vi "LSMcontroller_v56_from here for labview64bit.vi"() -> ()   [LabVIEW 2015] (continued)
                                n2126 = call "add channel to active arrayv2.vi"("line array in"=w5019, "line to add"=w5020) -> ("line array out"=w5018:u32[])  [unwired: 2 out]
                                n2127 = in-place-cluster #42("aDO"=w5018) -> (w5014:T12)
                                }
                                n2128 = call "2pparameters.vi"("Params in"=w5014, "command"="set") -> ()  [unwired: 1 out]
                                }
                                frame #1 {
                                n2129 = call "waveformparamsv2.vi"("command"="add DO", "add DO"=w5021) -> ()  [unwired: 3 in, 3 out]
                                }
                                frame #2 {
                                n2130 = call "waveformsDObuffer.vi"("command"="get") -> ("DO wf out"=w5026:digitalwaveform[])  [unwired: 1 in]
                                n2131 = Build Array (concatenate)(w5026, w5023) -> (w5025:digitalwaveform[])
                                n2132 = call "waveformsDObuffer.vi"("DO wf in"=w5025, "command"="set") -> ()  [unwired: 1 out]
                                }
                                }
                                }
                                frame 0 {
                                n2133 = stacked-sequence {
                                seq-local: [w5032 _ _] -> [_ w5042 w5059]
                                tunnel: w5031 -> [_ _ _]
                                tunnel: w5030 -> [_ _ _]
                                tunnel: w5029 -> [_ w5039 _]
                                tunnel: w5028 -> [_ _ w5058]
                                frame #0 {
                                n2134 = call "configuration.vi"("command"="get") -> ("config out"=w5037:T13)  [unwired: 2 in, 1 out]
                                n2135 = Unbundle By Name(w5037) -> ("LT timestamp"=w5033:u32)
                                n2136 = call "2pparameters.vi"("command"="get") -> ("params out"=w5036:T12)  [unwired: 1 in]
                                n2137 = Unbundle By Name(w5036) -> ("aDO"=w5034:u32[])
                                n2138 = Search 1D Array(1D array=w5034, element=w5033) -> (index of element=w5032:i32)  [unwired: 1 in]
                                }
                                frame #1 {
                                n2139 = local read "Measurement"() -> (w5041:T5)
                                n2140 = To Unsigned Long Integer(number=w5041) -> (unsigned 32bit integer=w5040:u32)
                                n2141 = case shown="5..7" w5040 {
                                tunnel: w5042 -> [_ w5046]
                                tunnel: w5039 -> [_ w5043]
                                frame 0..4, Default {
                                }
                                frame 5..7 {
                                n2142 = Index Array(array=w5043, index=0) -> (element=w5044:T20)
                                n2143 = call "waveformparamsv2.vi"("command"="get") -> ("Params out"=w5049:T16)  [unwired: 4 in, 2 out]
                                n2144 = in-place {
                                in-place-border: w5046 -> [w5053]
                                in-place-border: w5044 -> [w5051]
                                n2145 = in-place-cluster #43(w5049) -> ("DO parameters"=w5054:T19)
                                n2146 = in-place {
                                in-place-border: w5051 -> [w5055]
                                n2147 = in-place-array #44(w5054, w5053) -> ()  [unwired: 1 out]
                                n2148 = in-place-array #44(w5055) -> (w5052:T19)  [unwired: 1 out]
                                }
                                n2149 = in-place-cluster #43("DO parameters"=w5052) -> (w5047:T16)
                                }
                                n2150 = call "waveformparamsv2.vi"("command"="set", "Params in"=w5047) -> ()  [unwired: 3 in, 3 out]
                                }
                                }
                                }
                                frame #2 {
                                n2151 = local read "Measurement"() -> (w5057:T5)
                                n2152 = To Unsigned Long Integer(number=w5057) -> (unsigned 32bit integer=w5056:u32)
                                n2153 = case shown="5..7" w5056 {
                                tunnel: w5059 -> [_ w5063]
                                tunnel: w5058 -> [_ w5061]
                                frame 0..4, Default {
                                }
                                frame 5..7 {
                                n2154 = Index Array(array=w5061, index=0) -> (element=w5060:digitalwaveform)
                                n2155 = call "waveformsDObuffer.vi"("command"="get") -> ("DO wf out"=w5065:digitalwaveform[])  [unwired: 1 in]
                                n2156 = Replace Array Subset(array=w5065, new element=w5060, index=w5063) -> (w5067:digitalwaveform[])
                                n2157 = call "waveformsDObuffer.vi"("DO wf in"=w5067, "command"="set") -> ()  [unwired: 1 out]
                                }
                                }
                                }
                                }
                                }
                                }
                              }
                              frame #4 {
                                n2158 = call "Used AO lines.vi"() -> ("used AO names"=w5070:string[], "used AO lines"=w5068:tag[])  [unwired: 2 in]
                                n2159 = control-ref of="Analog Lines Plot"() -> (w5069:refnum<vi>)
                                n2160 = control-ref of="Digital Lines Plot"() -> (w5071:refnum<vi>)
                                n2161 = call "Used DO lines.vi"() -> ("used DO names"=w5072:string[], "used DO lines"=w5073:tag[])  [unwired: 2 in]
                                n2162 = local write "Analog Used Lines"(w5068) -> ()
                                n2163 = local write "Analog Used Names"(w5070) -> ()
                                n2164 = local write "Digital Used Lines"(w5073) -> ()
                                n2165 = local write "Digital Used Names"(w5072) -> ()
                                n2166 = call "prepDOWaveplot.vi"("DigitalGraph in"=w5071, "used DO names"=w5072) -> ()  [unwired: 1 in]
                                n2167 = call "prepAOWaveplot.vi"("WaveformGraph in"=w5069, "Analog Used Names"=w5070) -> ()  [unwired: 1 in]
                              }
                              frame #5 {
                                n2168 = local read "Meastab"() -> (w5088:enum32{"X-Y Image", "Linescan", "Timetrace"})
                                n2169 = property on="refwf" class="Ring (strict)"() -> ("RingText.Text"=w5085:string)  [unwired: 2 in, 2 out]
                                n2170 = case shown="\"Timetrace\"" w5088 {
                                tunnel: [w5090 w5091] -> w5089
                                frame "X-Y Image", Default {
                                n2171 = local read "Sampling rate"() -> (w5090:dbl)
                                }
                                frame "Timetrace" {
                                n2172 = local read "srateAODOtt"() -> (w5091:dbl)
                                }
                                }
                                n2173 = call "waveformsAObuffer.vi"("command"="get") -> ("AO wf out"=w5076:waveform(dbl)[])  [unwired: 1 in]
                                n2174 = local read "wavdet"() -> (w5086:bool)
                                n2175 = call "waveformsDObuffer.vi"("command"="get") -> ("DO wf out"=w5080:digitalwaveform[])  [unwired: 1 in]
                                n2176 = call "correctwaveformsizetemp.vi"("new sampling frequency (Hz)"=w5089, "start"=FALSE, "reference waveforms to"=w5085, "Analog waveforms in"=w5076, "stop"=TRUE, "Digital waveforms in"=w5080) -> ("analog wf out"=w5082:waveform(dbl)[], "Digital wf out"=w5084:digitalwaveform[], "measpoints"=w5087:i32)
                                n2177 = local write "Analog Lines Plot"(w5082) -> ()
                                n2178 = call "GetNumCamFramesv2.vi"("Digital Waveform Graph"=w5084) -> ("Numeric"=w5083:i32)  [unwired: 10 in]
                                n2179 = local write "Digital Lines Plot"(w5084) -> ()
                                n2180 = call "waveformsDObuffer.vi"("DO wf in"=w5084, "command"="set") -> ()  [unwired: 1 out]
                                n2181 = call "waveformsAObuffer.vi"("AO wf in"=w5082, "command"="set") -> ()  [unwired: 1 out]
                                n2182 = local write "Total Camera Frames"(w5083) -> ()
                                n2183 = case shown="True" w5086 {
                                tunnel: w5087 -> [_ w5092]
                                frame False {
                                }
                                frame True {
                                n2184 = local write "# of frames"(w5092) -> ()
                                }
                                }
                              }
                            }
                            n2185 = call "stoperaseCI.vi"() -> ()  [unwired: 12 in]
                            n2186 = call "stoperaseDO_img.vi"() -> ()  [unwired: 12 in]
                            n2187 = call "stoperaseAO_img.vi"() -> ()  [unwired: 12 in]
                            n2188 = call "stoperaseAI_img.vi"() -> ()  [unwired: 12 in]
                          }
                          frame #9 {
                            w5102 = FALSE ("Value (Signaling)")
                            n2189 = local read "save\ndata"() -> (w5097:bool)
                            n2190 = case shown="True" w5097 {
                              tunnel: w5096 -> [_ w5109]
                              frame False {
                              }
                              frame True {
                                n2191 = call "closebinaryfiles.vi"() -> ()  [unwired: 12 in]
                                n2192 = local read "filename prefix"() -> (w5111:string)
                                n2193 = local read "data dir"() -> (w5110:path)
                                n2194 = call "saveparams.vi"("timestamp"=w5109, "filename prefix in"=w5111, "data dir in"=w5110) -> ()  [unwired: 1 in]
                              }
                            }
                            n2195 = call "2pparameters.vi"("command"="get") -> ("params out"=w5093:T12)  [unwired: 1 in]
                            n2196 = Unbundle By Name(w5093) -> ("auto OD"=w5094:bool)
                            n2197 = case shown="True" w5094 {
                              frame False {
                              }
                              frame True {
                                n2198 = call "configuration.vi"("command"="get") -> ("config out"=w5105:T13)  [unwired: 2 in, 1 out]
                                n2199 = call "2pparameters.vi"("command"="get") -> ("params out"=w5108:T12)  [unwired: 1 in]
                                n2200 = Unbundle By Name(w5105) -> ("contour OD"=w5103:u16)
                                n2201 = Unbundle By Name(w5108) -> ("ODfilt"=w5104:u16)
                                n2202 = call "filterwheelcontrol_nothorlabslib.vi"("Current OD filt"=w5103, "New ODfilt"=w5104) -> ()  [unwired: 1 in]
                              }
                            }
                            n2203 = property on="Start" class="Bool (strict)"("Val(Sgnl)"=w5102) -> ()  [unwired: 2 in, 2 out]
                            n2204 = property on="Start" class="Bool (strict)"("Visible"=TRUE, "DisabledEnum"=T8."Enabled" ("Disabled")) -> ()  [unwired: 2 in, 2 out]
                            n2205 = property on="Stop" class="Bool (strict)"("Val(Sgnl)"=w5102) -> ()  [unwired: 2 in, 2 out]
                            n2206 = property on="Stop" class="Bool (strict)"("Visible"=FALSE, "DisabledEnum"=T8."Disabled" ("Disabled")) -> ()  [unwired: 2 in, 2 out]
                          }
                          frame #10 {
                            w5114 = T23 2 items=["no dialog", "OK message", "continue or stop message", "OK message + warnings", "continue/stop + warnings"] ("type of dialog (OK msg:1)")
                            n2207 = call "displayerrors.vi"() -> ("error IO"=w5115:errorcluster)
                            n2208 = call <vilib>:"General Error Handler.vi"("type of dialog (OK msg:1)"=w5114, "error in (no error)"=w5115) -> ("error out"=w5113:errorcluster)  [unwired: 9 in, 4 out]
                            n2209 = call <vilib>:"Clear Errors.vi"("error in (no error)"=w5113) -> ("error out"=w5112:errorcluster)  [unwired: 5 in, 1 out]
                            n2210 = call "seterrors.vi"("error IO"=w5112) -> ()
                          }
                        }
                      }
                    }
                  }
                  frame "Lifetime (point)" {
                    # "Disabled for conversion to 64 bit"
                    n2211 = disable-structure shown="Disabled" {
                      frame Disabled {
                        n2212 = stacked-sequence {
                          frame #0 {
                            w5126 = 12.5 ("x")
                            # "get from syncrate"
                            n2213 = local read "Bin size"() -> (w5120:T7)
                            n2214 = local read "Vx-ref"() -> (w5132:dbl)
                            n2215 = local read "Vy-ref"() -> (w5133:dbl)
                            n2216 = call "2pparameters.vi"("command"="get") -> ("params out"=w5118:T12)  [unwired: 1 in]
                            n2217 = Scale By Power Of 2(n=w5120, x=1.0 ("Y Scale.Range:Minimum")) -> (x*2^n=w5129:dbl)
                            n2218 = call "setposition.vi"("Vy"=w5133, "Vx"=w5132) -> ()  [unwired: 1 in]
                            n2219 = Unbundle By Name(w5118) -> ("autoshutter"=w5119:bool)
                            n2220 = Multiply(x=3000.0 ("Y Scale.Range:Minimum"), y=w5129) -> (x*y=w5127:dbl)
                            n2221 = Compound Arithmetic op=MULTIPLY(w5126, invert 3200.0 ("X Scale.Offset and Multiplier:Multiplier"), w5129) -> (w5128:dbl)
                            n2222 = case shown="True" w5119 {
                              frame False {
                              }
                              frame True {
                                n2223 = call "shuttercontrol.vi"("command"="open") -> ()  [unwired: 1 in, 1 out]
                              }
                            }
                            n2224 = call "lifetimeparameters.vi"("command"="get") -> ("Params out"=w5124:T21)  [unwired: 1 in]
                            n2225 = property on="Histogram" class="WFGraph (strict)"("XScale.Maximum"=w5126, "XScale.Minimum"=0.0 ("X Scale.Range:Minimum"), "YScale.Maximum"=w5127, "YScale.Minimum"=0.1 ("Y Scale.Range:Minimum"), "XScale.Multiplier"=w5128) -> ()  [unwired: 2 in, 2 out]
                            n2226 = Bundle By Name(cluster=w5124, "Bin size"=w5120) -> (w5125:T21)
                            n2227 = call "lifetimeparameters.vi"("Params in"=w5125, "command"="set") -> ()  [unwired: 1 out]
                            n2228 = property on="Histogram 2" class="WFGraph (strict)"("YScale.Maximum"=w5127, "XScale.Multiplier"=w5128, "XScale.Maximum"=w5126) -> ()  [unwired: 2 in, 2 out]
                            n2229 = call "2pparameters.vi"("command"="get") -> ("params out"=w5140:T12)  [unwired: 1 in]
                            n2230 = Bundle By Name(cluster=w5140, "type"="Lifetime (point)") -> (w5138:T12)
                            n2231 = property on="Stop" class="Bool (strict)"("Visible"=TRUE, "DisabledEnum"=T8."Enabled" ("Disabled")) -> ()  [unwired: 2 in, 2 out]
                            n2232 = property on="Start" class="Bool (strict)"("Visible"=FALSE, "DisabledEnum"=T8."Disabled and Grayed Out" ("Disabled")) -> ()  [unwired: 2 in, 2 out]
                            n2233 = call "2pparameters.vi"("Params in"=w5138, "command"="set") -> ()  [unwired: 1 out]
                          }
                          frame #1 {
                            n2234 = call "setup.vi"() -> ()  [unwired: 1 in]
                          }
                          frame #2 {
                            # "main loop"
                            n2235 = call "lifetimeparameters.vi"("command"="get") -> ("Params out"=w5150:T21)  [unwired: 1 in]
                            n2236 = Unbundle By Name(w5150) -> ("devidx"=w5148:i32)
                            n2237 = for {
                              N: 10000 -> [_]
                              tunnel: [w5151] -> w5146 mode=indexing
                              i -> [w5151]
                            }
                            n2238 = while {
                              tunnel: w5148 -> [w5155]
                              tunnel: w5146 -> [w5152]
                              i -> [w5153]
                              stop <- w5157 stop-if-true
                              n2239 = Increment(x=w5153) -> (x+1=w5154:i32)
                              n2240 = dll-call lib="phlib.dll" fn="_PH_GetCountRate@8" label="PH_GetCountRate"("devidx"=w5155, "channel"=0) -> (w5156:i32)  [unwired: 5 in, 2 out]
                              "SyncRate" <- w5156
                              n2241 = stacked-sequence {
                                seq-local: [_ _ w5164 _ _] -> [_ _ _ w5177 _]
                                seq-local: [_ _ w5163 _ _] -> [_ _ _ w5176 _]
                                seq-local: [_ w5161 _ _ _] -> [_ _ w5165 _ _]
                                tunnel: w5156 -> [_ _ _ w5184 _]
                                tunnel: w5152 -> [_ _ _ w5174 _]
                                frame #0 {
                                n2242 = call "start_binned.vi"() -> ()  [unwired: 1 in]
                                }
                                frame #1 {
                                n2243 = call "get-histogram.vi"() -> ("IntegralCount"=→"Integral count":u32, "Histogram"=w5161:u32[])
                                "Histogram" <- w5161
                                }
                                frame #2 {
                                n2244 = Search 1D Array(1D array=w5165, element=u32 0) -> (index of element=w5163:i32)  [unwired: 1 in]
                                n2245 = Multiply(x=w5163, y=0.99) -> (x*y=w5169:dbl)
                                n2246 = Array Subset(array=w5165, index=0, length=w5169) -> (w5172:u32[])
                                n2247 = Array Max & Min(array=w5172) -> (max index (indices)=w5166:i32)  [unwired: 3 out]
                                n2248 = Split 1D Array(array=w5172, index=w5166) -> (second subarray=w5168:u32[])  [unwired: 1 out]
                                n2249 = Array Max & Min(array=w5168) -> (min index (indices)=w5167:i32)  [unwired: 3 out]
                                n2250 = Split 1D Array(array=w5168, index=w5167) -> (first subarray=w5164:u32[])  [unwired: 1 out]
                                "Histogram 2" <- w5164
                                }
                                frame #3 {
                                n2251 = Array Size(array=w5177) -> (size(s)=w5179:i32)
                                n2252 = Array Subset(array=w5174, index=0, length=w5179) -> (w5178:i32[])
                                n2253 = Compound Arithmetic op=MULTIPLY(1000000000.0 ("value"), invert w5184, invert w5176, w5178) -> (w5175:dbl[])
                                n2254 = call <vilib>:"Exponential Fit.vi"("Y"=w5177, "X"=w5175) -> ("damping"=w5181:dbl)  [unwired: 8 in, 5 out]
                                n2255 = Divide(x=-1.0 ("y"), y=w5181) -> (x/y=→"Lifetime (ns)":dbl)
                                }
                                frame #4 {
                                n2256 = local read "downright"() -> (w5191:bool)
                                n2257 = local read "downleft"() -> (w5193:bool)
                                n2258 = local read "upright"() -> (w5189:bool)
                                n2259 = local read "upleft"() -> (w5187:bool)
                                n2260 = local read "down"() -> (w5192:bool)
                                n2261 = local read "right"() -> (w5190:bool)
                                n2262 = local read "left"() -> (w5194:bool)
                                n2263 = local read "up"() -> (w5188:bool)
                                n2264 = Compound Arithmetic op=OR(w5187, w5188, w5189, w5190, w5191, w5192, w5193, w5194) -> (w5186:bool)
                                n2265 = case shown="True" w5186 {
                                frame False {
                                }
                                frame True {
                                n2266 = stacked-sequence {
                                frame #0 {
                                n2267 = local read "downright"() -> (w5196:bool)
                                n2268 = local read "downleft"() -> (w5198:bool)
                                n2269 = local read "BigSmall"() -> (w5195:bool)
                                n2270 = local read "upright"() -> (w5200:bool)
                                n2271 = local read "upleft"() -> (w5203:bool)
                                n2272 = local read "down"() -> (w5199:bool)
                                n2273 = local read "right"() -> (w5201:bool)
                                n2274 = local read "left"() -> (w5197:bool)
                                n2275 = local read "up"() -> (w5202:bool)
                                n2276 = call "movestageparams.vi"("command"="get") -> ("Params out"=w5206:T22)  [unwired: 1 in]
                                n2277 = Bundle By Name(cluster=w5206, "upleft"=w5203, "up"=w5202, "upright"=w5200, "right"=w5201, "downright"=w5196, "down"=w5199, "downleft"=w5198, "left"=w5197, "Bigsmall"=w5195) -> (w5207:T22)
                                n2278 = call "movestageparams.vi"("Params in"=w5207, "command"="set") -> ()  [unwired: 1 out]
                                }
                                frame #1 {
                                n2279 = call "movestage.vi"() -> ()  [unwired: 12 in]
                                }
                                frame #2 {
                                w5208 = FALSE ("OK Button")
                                w5209 = FALSE ("OK Button")
                                n2280 = property on="down" class="Bool (strict)"("Value"=w5209) -> ()  [unwired: 2 in, 2 out]
                                n2281 = property on="up" class="Bool (strict)"("Value"=w5209) -> ()  [unwired: 2 in, 2 out]
                                n2282 = property on="right" class="Bool (strict)"("Value"=w5209) -> ()  [unwired: 2 in, 2 out]
                                n2283 = property on="left" class="Bool (strict)"("Value"=w5209) -> ()  [unwired: 2 in, 2 out]
                                n2284 = property on="upleft" class="Bool (strict)"("Value"=w5208) -> ()  [unwired: 2 in, 2 out]
                                n2285 = property on="upright" class="Bool (strict)"("Value"=w5208) -> ()  [unwired: 2 in, 2 out]
                                n2286 = property on="downleft" class="Bool (strict)"("Value"=w5208) -> ()  [unwired: 2 in, 2 out]
                                n2287 = property on="downright" class="Bool (strict)"("Value"=w5208) -> ()  [unwired: 2 in, 2 out]
                                }
                                }
                                }
                                }
                                }
                              }
                              n2288 = dll-call lib="phlib.dll" fn="_PH_GetCountRate@8" label="PH_GetCountRate"("devidx"=w5155, "channel"=1) -> (→"Ch1Rate":i32)  [unwired: 5 in, 2 out]
                              n2289 = local read "Stop"() -> (w5157:bool)
                              n2290 = local write "points recorded"(w5154) -> ()
                            }
                          }
                          frame #3 {
                            w5217 = FALSE ("Value (Signaling)")
                            n2291 = call "2pparameters.vi"("command"="get") -> ("params out"=w5211:T12)  [unwired: 1 in]
                            n2292 = Unbundle By Name(w5211) -> ("autoshutter"=w5212:bool)
                            n2293 = case shown="True" w5212 {
                              frame False {
                              }
                              frame True {
                                n2294 = call "shuttercontrol.vi"("command"="close") -> ()  [unwired: 1 in, 1 out]
                              }
                            }
                            n2295 = property on="Start" class="Bool (strict)"("Val(Sgnl)"=w5217) -> ()  [unwired: 2 in, 2 out]
                            n2296 = property on="Start" class="Bool (strict)"("Visible"=TRUE, "DisabledEnum"=T8."Enabled" ("Disabled")) -> ()  [unwired: 2 in, 2 out]
                            n2297 = property on="Stop" class="Bool (strict)"("Val(Sgnl)"=w5217) -> ()  [unwired: 2 in, 2 out]
                            n2298 = property on="Stop" class="Bool (strict)"("Visible"=FALSE, "DisabledEnum"=T8."Disabled" ("Disabled")) -> ()  [unwired: 2 in, 2 out]
                          }
                        }
                      }
                      frame Enabled {
                      }
                    }
                    n2299 = local write "64bit disabled"(TRUE ("64bit disabled")) -> ()
                  }
                }
              }
            }
          }
          event "avpp", "Angle ref", "xpixels ref", "Vx-min ref", "Vx-max ref", "ypixels ref", "Vy-min ref", "Vy-max ref", "ROI Type", "Sampling rate": Value Change {
            n2300 = event-data() -> ()  [unwired: 1 in, 6 out]
            n2301 = local read "avpp"() -> (w5236:i32)
            n2302 = local read "Angle ref"() -> (w5235:dbl)
            n2303 = local read "ROI Type"() -> (w5234:u16)
            n2304 = local read "xpixels ref"() -> (w5231:i32)
            n2305 = local read "Vx-min ref"() -> (w5230:dbl)
            n2306 = local read "Vx-max ref"() -> (w5229:dbl)
            n2307 = local read "ypixels ref"() -> (w5227:i32)
            n2308 = local read "Vy-min ref"() -> (w5228:dbl)
            n2309 = local read "Vy-max ref"() -> (w5224:dbl)
            n2310 = local read "Sampling rate"() -> (w5219:dbl)
            n2311 = local read "# of frames"() -> (w5223:i32)
            n2312 = local read "maxbufferAI"() -> (w5222:i32)
            n2313 = local read "Override AI buffer"() -> (w5220:bool)
            n2314 = call "2pparameters.vi"("command"="get") -> ("params out"=w5233:T12)  [unwired: 1 in]
            n2315 = Bundle By Name(cluster=w5233, "avpp"=w5236, "Angle Img"=w5235, "Xpixels Img"=w5231, "Vx-min Img"=w5230, "VX-max Img"=w5229, "Ypixels Img"=w5227, "Vy-min Img"=w5228, "Vy-max Img"=w5224, "srate"=w5219, "srate Img"=w5219, "measpoints"=w5223, "maxbufferAI"=w5222, "Drawing Mode"=w5234, "Vz-reset"=0.0, "AIoverride"=w5220) -> (w5225:T12)
            n2316 = call "2pparameters.vi"("Params in"=w5225, "command"="set") -> ()  [unwired: 1 out]
          }
          event "# of frames": Value Change {
            n2317 = event-data() -> ()  [unwired: 1 in, 6 out]
            n2318 = local read "Meastab"() -> (w5237:enum32{"X-Y Image", "Linescan", "Timetrace"})
            n2319 = case shown="\"X-Y Image\", Default" w5237 {
              frame "X-Y Image", Default {
                n2320 = local read "# of frames"() -> (w5238:i32)
                n2321 = call "2pparameters.vi"("command"="get") -> ("params out"=w5242:T12)  [unwired: 1 in]
                n2322 = Bundle By Name(cluster=w5242, "measpoints"=w5238) -> (w5239:T12)
                n2323 = call "2pparameters.vi"("Params in"=w5239, "command"="set") -> ()  [unwired: 1 out]
              }
              frame "Linescan" {
                n2324 = local read "srateAODOtt"() -> (w5252:dbl)
                n2325 = local read "# of frames"() -> (w5248:i32)
                n2326 = local read "refreshtime"() -> (w5254:dbl)
                n2327 = local read "bin"() -> (w5249:dbl)
                n2328 = call "tt_timeandsamples.vi"("bin"=w5249, "refreshtime"=w5254, "srateAODOtt"=w5252, "tot#ofsamples"=w5248) -> ("refreshrate"=w5251:dbl, "refreshbuffer"=w5250:i32, "timetracecycles"=w5247:i32)  [unwired: 5 in]
                n2329 = call "2pparameters.vi"("command"="get") -> ("params out"=w5244:T12)  [unwired: 1 in]
                n2330 = Bundle By Name(cluster=w5244, "measpoints"=w5248, "tt_cycles"=w5247, "refreshbuffer"=w5250, "refreshrate"=w5251) -> (w5246:T12)
                n2331 = Reciprocal(x=w5251) -> (1/x=w5253:dbl)
                n2332 = local write "refreshtime"(w5253) -> ()
                n2333 = call "2pparameters.vi"("Params in"=w5246, "command"="set") -> ()  [unwired: 1 out]
              }
              frame "Timetrace" {
                n2334 = local read "srateAODOtt"() -> (w5264:dbl)
                n2335 = local read "# of frames"() -> (w5260:i32)
                n2336 = local read "refreshtime"() -> (w5266:dbl)
                n2337 = local read "bin"() -> (w5261:dbl)
                n2338 = call "tt_timeandsamples.vi"("bin"=w5261, "refreshtime"=w5266, "srateAODOtt"=w5264, "tot#ofsamples"=w5260) -> ("refreshrate"=w5263:dbl, "refreshbuffer"=w5262:i32, "timetracecycles"=w5259:i32)  [unwired: 5 in]
                n2339 = call "2pparameters.vi"("command"="get") -> ("params out"=w5256:T12)  [unwired: 1 in]
                n2340 = Bundle By Name(cluster=w5256, "measpoints"=w5260, "tt_cycles"=w5259, "refreshbuffer"=w5262, "refreshrate"=w5263) -> (w5258:T12)
                n2341 = Reciprocal(x=w5263) -> (1/x=w5265:dbl)
                n2342 = local write "refreshtime"(w5265) -> ()
                n2343 = call "2pparameters.vi"("Params in"=w5258, "command"="set") -> ()  [unwired: 1 out]
              }
            }
          }
          event "srateAODOtt", "refreshtime", "Vx-ref", "Vy-ref", "Vx-min draw", "Vx-max draw", "Vy-min draw", "Vy-max draw", "bin": Value Change {
            n2344 = event-data() -> ()  [unwired: 1 in, 6 out]
            n2345 = local read "ypixels ref"() -> (w5298:i32)
            n2346 = local read "Vy-min draw"() -> (w5274:dbl)
            n2347 = local read "Vy-max draw"() -> (w5273:dbl)
            n2348 = local read "Vx-min draw"() -> (w5276:dbl)
            n2349 = local read "Vx-max draw"() -> (w5275:dbl)
            n2350 = local read "xpixels ref"() -> (w5272:i32)
            n2351 = local read "ROI Type"() -> (w5271:u16)
            n2352 = local read "Pel"() -> (w5270:dbl)
            n2353 = local read "srateAODOtt"() -> (w5280:dbl)
            n2354 = local read "# of frames"() -> (w5285:i32)
            n2355 = local read "refreshtime"() -> (w5278:dbl)
            n2356 = local read "bin"() -> (w5283:dbl)
            n2357 = local read "Override AI buffer"() -> (w5268:bool)
            n2358 = local read "finite samples"() -> (w5292:bool)
            n2359 = local read "srateAODOtt"() -> (w5267:dbl)
            n2360 = local read "srateAODOtt"() -> (w5286:dbl)
            n2361 = local read "continuous"() -> (w5291:bool)
            n2362 = local read "Angle ref"() -> (w5277:dbl)
            n2363 = local read "wavdet"() -> (w5293:bool)
            n2364 = local read "Vx-ref"() -> (w5288:dbl)
            n2365 = local read "Vy-ref"() -> (w5290:dbl)
            n2366 = local read "avpp"() -> (w5289:i32)
            n2367 = call "tt_timeandsamples.vi"("bin"=w5283, "refreshtime"=w5278, "srateAODOtt"=w5280, "tot#ofsamples"=w5285) -> ("refreshrate"=w5281:dbl, "refreshbuffer"=w5282:i32, "timetracecycles"=w5287:i32)  [unwired: 5 in]
            n2368 = local read "bin"() -> (w5284:dbl)
            n2369 = call "2pparameters.vi"("command"="get") -> ("params out"=w5296:T12)  [unwired: 1 in]
            n2370 = Bundle By Name(cluster=w5296, "Drawing Mode"=w5271, "measpoints"=w5285, "tt_cycles"=w5287, "refreshbuffer"=w5282, "refreshrate"=w5281, "Vx-ref"=w5288, "Vy-ref"=w5290, "srate"=w5267, "finite"=w5292, "cont"=w5291, "wavdet"=w5293, "avpp"=w5289, "srateAODO"=w5286, "bufferAI"=w5282, "bin"=w5284, "Angle Img"=w5277, "Vxminref"=w5276, "Vxmaxref"=w5275, "Vyminref"=w5274, "Vymaxref"=w5273, "Xpixels Img"=w5272, "Ypixels Img"=w5298, "Pel"=w5270, "Vz-reset"=0.0, "AIoverride"=w5268) -> (w5294:T12)
            n2371 = Reciprocal(x=w5281) -> (1/x=w5279:dbl)
            n2372 = local write "refreshtime"(w5279) -> ()
            n2373 = call "2pparameters.vi"("Params in"=w5294, "command"="set") -> ()  [unwired: 1 out]
          }
          event "Init": Value Change {
            # "Disabled for conversion to 64 bit"
            n2374 = event-data() -> ()  [unwired: 1 in, 6 out]
            n2375 = disable-structure shown="Disabled" {
              frame Disabled {
                n2376 = flat-sequence {
                  frame #0 {
                    n2377 = local read "Measurement"() -> (w5300:T5)
                    n2378 = case shown="\"Lifetime (scan)\", \"Lifetime (contour)\"" w5300 {
                      frame "X-Y-t movie", Default {
                      }
                      frame "Lifetime (point)" {
                        n2379 = stacked-sequence {
                          frame #0 {
                            n2380 = call "initialize.vi"("mode"=0) -> ()
                          }
                          frame #1 {
                            n2381 = call "calib.vi"() -> ()  [unwired: 1 in]
                          }
                        }
                      }
                      frame "Lifetime (scan)", "Lifetime (contour)" {
                        n2382 = stacked-sequence {
                          frame #0 {
                            n2383 = call "initialize.vi"("mode"=3) -> ()
                          }
                          frame #1 {
                            n2384 = call "calib.vi"() -> ()  [unwired: 1 in]
                          }
                        }
                      }
                    }
                  }
                  frame #1 {
                    n2385 = property on="Start" class="Bool (strict)"("Visible"=TRUE, "DisabledEnum"=T8."Enabled" ("Disabled")) -> ()  [unwired: 2 in, 2 out]
                    n2386 = property on="Init" class="Bool (strict)"("Visible"=FALSE, "DisabledEnum"=T8."Disabled and Grayed Out" ("Disabled"), "Value"=FALSE ("Init")) -> ()  [unwired: 2 in, 2 out]
                  }
                }
              }
              frame Enabled {
              }
            }
            n2387 = local write "64bit disabled"(TRUE ("64bit disabled")) -> ()
          }
          event "Measurement": Value Change {
            n2388 = event-data() -> ()  [unwired: 1 in, 5 out]
            n2389 = case shown="\"Lifetime (contour)\"" "Measurement" {
              frame "X-Y-t movie" {
                w5310 = T8."Disabled" ("Disabled")
                w5309 = FALSE ("Visible")
                n2390 = call "2pparameters.vi"("command"="get") -> ("params out"=w5320:T12)  [unwired: 1 in]
                n2391 = local write "graphtab"(T6."image" ("graphtab")) -> ()
                n2392 = local write "Save tab"(enum32{"withsave", "withoutsave"}."withsave" ("Save tab")) -> ()
                n2393 = Bundle By Name(cluster=w5320, "type"="X-Y-t movie") -> (w5318:T12)
                n2394 = call "2pparameters.vi"("Params in"=w5318, "command"="set") -> ()  [unwired: 1 out]
                n2395 = property on="refreshtime" class="DigNum (strict)"("Visible"=FALSE, "DisabledEnum"=T8."Disabled and Grayed Out" ("Disabled")) -> ()  [unwired: 2 in, 2 out]
                n2396 = property on="ttt" class="Enum (strict)"("Visible"=FALSE) -> ()  [unwired: 2 in, 2 out]
                n2397 = property on="# of frames" class="DigNum (strict)"("DisabledEnum"=T8."Enabled" ("Disabled"), "Caption.Text"="# of frames") -> ()  [unwired: 2 in, 2 out]
                n2398 = property on="continuous" class="Bool (strict)"("Visible"=TRUE, "DisabledEnum"=T8."Enabled" ("Disabled")) -> ()  [unwired: 2 in, 2 out]
                n2399 = property on="finite samples" class="Bool (strict)"("Visible"=TRUE, "DisabledEnum"=T8."Enabled" ("Disabled")) -> ()  [unwired: 2 in, 2 out]
                n2400 = property on="avpp" class="DigNum (strict)"("Visible"=TRUE, "DisabledEnum"=T8."Enabled" ("Disabled")) -> ()  [unwired: 2 in, 2 out]
                n2401 = property on="srateAODOtt" class="DigNum (strict)"("Visible"=FALSE, "DisabledEnum"=T8."Disabled" ("Disabled")) -> ()  [unwired: 2 in, 2 out]
                n2402 = local write "save\ndata"(TRUE ("save\ndata")) -> ()
                n2403 = property on="finite samples" class="Bool (strict)"("Val(Sgnl)"=TRUE ("continuous for display")) -> ()  [unwired: 2 in, 2 out]
                n2404 = property on="continuous" class="Bool (strict)"("Value"=FALSE ("continuous for display")) -> ()  [unwired: 2 in, 2 out]
                n2405 = property on="Current Average" class="DigNum (strict)"("Visible"=TRUE, "DisabledEnum"=T8."Enabled" ("Disabled")) -> ()  [unwired: 2 in, 2 out]
                n2406 = property on="img_CH1" class="IntGraph (strict)"("ZScale.Maximum"=7.0 ("Z Scale.Range:Maximum")) -> ()  [unwired: 2 in, 2 out]
                n2407 = property on="Sampling rate" class="DigNum (strict)"("Visible"=TRUE, "DisabledEnum"=T8."Enabled" ("Disabled")) -> ()  [unwired: 2 in, 2 out]
                n2408 = property on="Pel" class="DigNum (strict)"("Visible"=w5309, "DisabledEnum"=w5310) -> ()  [unwired: 2 in, 2 out]
                n2409 = property on="bin" class="DigNum (strict)"("Visible"=w5309, "DisabledEnum"=w5310) -> ()  [unwired: 2 in, 2 out]
                "Meastab" <- enum32{"X-Y Image", "Linescan", "Timetrace"}."X-Y Image" ("Meastab")
                "Zscantab" <- enum32{"withzscan", "withoutzscan", "lifetime"}."withoutzscan" ("Zscantab")
              }
              frame "X-Y-Z stack" {
                w5342 = T8."Disabled" ("Disabled")
                w5341 = FALSE ("Visible")
                n2410 = call "2pparameters.vi"("command"="get") -> ("params out"=w5352:T12)  [unwired: 1 in]
                n2411 = call "2pparameters.vi"("command"="get") -> ("params out"=w5356:T12)  [unwired: 1 in]
                n2412 = Bundle By Name(cluster=w5352, "type"="X-Y-Z stack") -> (w5350:T12)
                n2413 = Unbundle By Name(w5356) -> ("motorref"=w5355:refnum<k7>)
                n2414 = call "2pparameters.vi"("Params in"=w5350, "command"="set") -> ()  [unwired: 1 out]
                n2415 = local write "Zscantab"(enum32{"withzscan", "withoutzscan", "lifetime"}."withzscan" ("Zscantab")) -> ()
                n2416 = local write "Meastab"(enum32{"X-Y Image", "Linescan", "Timetrace"}."X-Y Image" ("Meastab")) -> ()
                n2417 = invoke class="MG17Motor" method="GetPosition"(reference=w5355, "lChanID"=0, "pfPosition"=sgl 0.0) -> ("pfPosition"=w5367:sgl)  [unwired: 2 in, 4 out]
                n2418 = property on="refreshtime" class="DigNum (strict)"("Visible"=FALSE, "DisabledEnum"=T8."Disabled and Grayed Out" ("Disabled")) -> ()  [unwired: 2 in, 2 out]
                n2419 = property on="ttt" class="Enum (strict)"("Visible"=FALSE) -> ()  [unwired: 2 in, 2 out]
                n2420 = Multiply(x=w5367, y=1000.0) -> (x*y=w5366:dbl)
                n2421 = local write "Actual Z position"(w5366) -> ()
                n2422 = local write "Save tab"(enum32{"withsave", "withoutsave"}."withsave" ("Save tab")) -> ()
                n2423 = property on="finite samples" class="Bool (strict)"("Visible"=FALSE, "DisabledEnum"=T8."Disabled and Grayed Out" ("Disabled")) -> ()  [unwired: 2 in, 2 out]
                n2424 = property on="avpp" class="DigNum (strict)"("Visible"=TRUE, "DisabledEnum"=T8."Enabled" ("Disabled")) -> ()  [unwired: 2 in, 2 out]
                n2425 = property on="continuous" class="Bool (strict)"("Visible"=FALSE, "DisabledEnum"=T8."Disabled and Grayed Out" ("Disabled")) -> ()  [unwired: 2 in, 2 out]
                n2426 = property on="img_CH1" class="IntGraph (strict)"("ZScale.Maximum"=7.0 ("Z Scale.Range:Maximum")) -> ()  [unwired: 2 in, 2 out]
                n2427 = property on="srateAODOtt" class="DigNum (strict)"("Visible"=FALSE, "DisabledEnum"=T8."Disabled" ("Disabled")) -> ()  [unwired: 2 in, 2 out]
                n2428 = property on="Pel" class="DigNum (strict)"("Visible"=w5341, "DisabledEnum"=w5342) -> ()  [unwired: 2 in, 2 out]
                n2429 = property on="bin" class="DigNum (strict)"("Visible"=w5341, "DisabledEnum"=w5342) -> ()  [unwired: 2 in, 2 out]
                n2430 = property on="Current Average" class="DigNum (strict)"("Visible"=TRUE, "DisabledEnum"=T8."Enabled" ("Disabled")) -> ()  [unwired: 2 in, 2 out]
                n2431 = property on="# of frames" class="DigNum (strict)"("Caption.Text"="# of slices", "DisabledEnum"=T8."Disabled and Grayed Out" ("Disabled")) -> ()  [unwired: 2 in, 2 out]
                n2432 = local write "save\ndata"(TRUE ("save\ndata")) -> ()
                n2433 = property on="finite samples" class="Bool (strict)"("Val(Sgnl)"=TRUE ("continuous for display")) -> ()  [unwired: 2 in, 2 out]
                n2434 = property on="continuous" class="Bool (strict)"("Value"=FALSE ("continuous for display")) -> ()  [unwired: 2 in, 2 out]
                n2435 = property on="Sampling rate" class="DigNum (strict)"("Visible"=TRUE, "DisabledEnum"=T8."Enabled" ("Disabled")) -> ()  [unwired: 2 in, 2 out]
              }
              frame "X-Y-Z-t movie" {
                w5381 = T8."Disabled" ("Disabled")
                w5380 = FALSE ("Visible")
                n2436 = property on="# of frames" class="DigNum (strict)"("DisabledEnum"=T8."Enabled" ("Disabled")) -> ()  [unwired: 2 in, 2 out]
                n2437 = property on="Current Average" class="DigNum (strict)"("Visible"=TRUE, "DisabledEnum"=T8."Enabled" ("Disabled")) -> ()  [unwired: 2 in, 2 out]
                n2438 = property on="avpp" class="DigNum (strict)"("Visible"=TRUE, "DisabledEnum"=T8."Enabled" ("Disabled")) -> ()  [unwired: 2 in, 2 out]
                n2439 = local write "Save tab"(enum32{"withsave", "withoutsave"}."withsave" ("Save tab")) -> ()
                n2440 = local write "Zscantab"(enum32{"withzscan", "withoutzscan", "lifetime"}."withzscan" ("Zscantab")) -> ()
                n2441 = local write "Meastab"(enum32{"X-Y Image", "Linescan", "Timetrace"}."X-Y Image" ("Meastab")) -> ()
                n2442 = property on="refreshtime" class="DigNum (strict)"("Visible"=FALSE, "DisabledEnum"=T8."Disabled and Grayed Out" ("Disabled")) -> ()  [unwired: 2 in, 2 out]
                n2443 = property on="ttt" class="Enum (strict)"("Visible"=FALSE) -> ()  [unwired: 2 in, 2 out]
                n2444 = call "2pparameters.vi"("command"="get") -> ("params out"=w5391:T12)  [unwired: 1 in]
                n2445 = Bundle By Name(cluster=w5391, "type"="X-Y-Z-t movie") -> (w5389:T12)
                n2446 = property on="continuous" class="Bool (strict)"("Visible"=TRUE, "DisabledEnum"=T8."Enabled" ("Disabled")) -> ()  [unwired: 2 in, 2 out]
                n2447 = property on="finite samples" class="Bool (strict)"("Visible"=TRUE, "DisabledEnum"=T8."Enabled" ("Disabled")) -> ()  [unwired: 2 in, 2 out]
                n2448 = call "2pparameters.vi"("Params in"=w5389, "command"="set") -> ()  [unwired: 1 out]
                n2449 = property on="srateAODOtt" class="DigNum (strict)"("Visible"=FALSE, "DisabledEnum"=T8."Disabled" ("Disabled")) -> ()  [unwired: 2 in, 2 out]
                n2450 = local write "save\ndata"(TRUE ("save\ndata")) -> ()
                n2451 = property on="img_CH1" class="IntGraph (strict)"("ZScale.Maximum"=7.0 ("Z Scale.Range:Maximum")) -> ()  [unwired: 2 in, 2 out]
                n2452 = property on="continuous" class="Bool (strict)"("Value"=FALSE ("continuous for display")) -> ()  [unwired: 2 in, 2 out]
                n2453 = property on="finite samples" class="Bool (strict)"("Value"=TRUE ("continuous for display")) -> ()  [unwired: 2 in, 2 out]
                n2454 = property on="Sampling rate" class="DigNum (strict)"("Visible"=TRUE, "DisabledEnum"=T8."Enabled" ("Disabled")) -> ()  [unwired: 2 in, 2 out]
                n2455 = property on="Pel" class="DigNum (strict)"("Visible"=w5380, "DisabledEnum"=w5381) -> ()  [unwired: 2 in, 2 out]
                n2456 = property on="bin" class="DigNum (strict)"("Visible"=w5380, "DisabledEnum"=w5381) -> ()  [unwired: 2 in, 2 out]
              }
              frame "linescan" {
                w5411 = T8."Enabled" ("Disabled")
                w5410 = TRUE ("Visible")
                w5413 = T8."Enabled" ("Disabled")
                w5412 = TRUE ("Visible")
                n2457 = local write "Meastab"(enum32{"X-Y Image", "Linescan", "Timetrace"}."Linescan" ("Meastab")) -> ()
                n2458 = property on="Current Average" class="DigNum (strict)"("Visible"=TRUE, "DisabledEnum"=T8."Enabled" ("Disabled")) -> ()  [unwired: 2 in, 2 out]
                n2459 = local write "Save tab"(enum32{"withsave", "withoutsave"}."withsave" ("Save tab")) -> ()
                n2460 = local write "Zscantab"(enum32{"withzscan", "withoutzscan", "lifetime"}."withoutzscan" ("Zscantab")) -> ()
                n2461 = property on="refreshtime" class="DigNum (strict)"("Visible"=FALSE, "DisabledEnum"=T8."Disabled and Grayed Out" ("Disabled")) -> ()  [unwired: 2 in, 2 out]
                n2462 = property on="continuous" class="Bool (strict)"("Value"=FALSE ("continuous for display")) -> ()  [unwired: 2 in, 2 out]
                n2463 = property on="finite samples" class="Bool (strict)"("Value"=TRUE ("continuous for display")) -> ()  [unwired: 2 in, 2 out]
                n2464 = property on="ttt" class="Enum (strict)"("Visible"=FALSE) -> ()  [unwired: 2 in, 2 out]
                n2465 = local write "save\ndata"(TRUE ("save\ndata")) -> ()
                n2466 = call "2pparameters.vi"("command"="get") -> ("params out"=w5422:T12)  [unwired: 1 in]
                n2467 = Bundle By Name(cluster=w5422, "type"="linescan") -> (w5420:T12)
                n2468 = property on="# of frames" class="DigNum (strict)"("DisabledEnum"=T8."Enabled" ("Disabled"), "Caption.Text"="# of lines") -> ()  [unwired: 2 in, 2 out]
                n2469 = property on="continuous" class="Bool (strict)"("Visible"=TRUE, "DisabledEnum"=T8."Enabled" ("Disabled")) -> ()  [unwired: 2 in, 2 out]
                n2470 = property on="avpp" class="DigNum (strict)"("Visible"=TRUE, "DisabledEnum"=T8."Enabled" ("Disabled")) -> ()  [unwired: 2 in, 2 out]
                n2471 = property on="finite samples" class="Bool (strict)"("Visible"=TRUE, "DisabledEnum"=T8."Enabled" ("Disabled")) -> ()  [unwired: 2 in, 2 out]
                n2472 = property on="srateAODOtt" class="DigNum (strict)"("Visible"=TRUE, "DisabledEnum"=T8."Enabled" ("Disabled")) -> ()  [unwired: 2 in, 2 out]
                n2473 = call "2pparameters.vi"("Params in"=w5420, "command"="set") -> ()  [unwired: 1 out]
                n2474 = property on="Pel" class="DigNum (strict)"("Visible"=w5412, "DisabledEnum"=w5413) -> ()  [unwired: 2 in, 2 out]
                n2475 = property on="bin" class="DigNum (strict)"("Visible"=w5412, "DisabledEnum"=w5413) -> ()  [unwired: 2 in, 2 out]
                n2476 = property on="Sampling rate" class="DigNum (strict)"("Visible"=FALSE, "DisabledEnum"=T8."Disabled" ("Disabled")) -> ()  [unwired: 2 in, 2 out]
                n2477 = property on="Pel" class="DigNum (strict)"("Visible"=w5410, "DisabledEnum"=w5411) -> ()  [unwired: 2 in, 2 out]
                n2478 = property on="bin" class="DigNum (strict)"("Visible"=w5410, "DisabledEnum"=w5411) -> ()  [unwired: 2 in, 2 out]
              }
              frame "Timetrace" {
                w5443 = T8."Enabled" ("Disabled")
                w5442 = TRUE ("Visible")
                n2479 = call "2pparameters.vi"("command"="get") -> ("params out"=w5448:T12)  [unwired: 1 in]
                n2480 = local write "Meastab"(enum32{"X-Y Image", "Linescan", "Timetrace"}."Timetrace" ("Meastab")) -> ()
                n2481 = Unbundle By Name(w5448) -> ("Angle draw"=w5450:dbl)
                n2482 = local write "Zscantab"(enum32{"withzscan", "withoutzscan", "lifetime"}."withoutzscan" ("Zscantab")) -> ()
                n2483 = property on="# of frames" class="DigNum (strict)"("DisabledEnum"=T8."Enabled" ("Disabled"), "Caption.Text"="# of samples") -> ()  [unwired: 2 in, 2 out]
                n2484 = property on="refreshtime" class="DigNum (strict)"("Visible"=TRUE, "DisabledEnum"=T8."Enabled" ("Disabled")) -> ()  [unwired: 2 in, 2 out]
                n2485 = property on="avpp" class="DigNum (strict)"("Visible"=FALSE, "DisabledEnum"=T8."Disabled and Grayed Out" ("Disabled")) -> ()  [unwired: 2 in, 2 out]
                n2486 = property on="Current Average" class="DigNum (strict)"("Visible"=FALSE, "DisabledEnum"=T8."Disabled and Grayed Out" ("Disabled")) -> ()  [unwired: 2 in, 2 out]
                n2487 = local write "Angle drawing"(w5450) -> ()
                n2488 = property on="ttt" class="Enum (strict)"("Visible"=TRUE) -> ()  [unwired: 2 in, 2 out]
                n2489 = property on="continuous" class="Bool (strict)"("Visible"=TRUE, "DisabledEnum"=T8."Enabled" ("Disabled")) -> ()  [unwired: 2 in, 2 out]
                n2490 = property on="finite samples" class="Bool (strict)"("Visible"=TRUE, "DisabledEnum"=T8."Enabled" ("Disabled")) -> ()  [unwired: 2 in, 2 out]
                n2491 = local write "save\ndata"(TRUE ("save\ndata")) -> ()
                n2492 = property on="finite samples" class="Bool (strict)"("Val(Sgnl)"=TRUE ("continuous for display")) -> ()  [unwired: 2 in, 2 out]
                n2493 = property on="continuous" class="Bool (strict)"("Value"=FALSE ("continuous for display")) -> ()  [unwired: 2 in, 2 out]
                n2494 = local write "Save tab"(enum32{"withsave", "withoutsave"}."withsave" ("Save tab")) -> ()
                n2495 = property on="srateAODOtt" class="DigNum (strict)"("Visible"=TRUE, "DisabledEnum"=T8."Enabled" ("Disabled")) -> ()  [unwired: 2 in, 2 out]
                n2496 = call "2pparameters.vi"("command"="get") -> ("params out"=w5455:T12)  [unwired: 1 in]
                n2497 = Bundle By Name(cluster=w5455, "type"="Timetrace") -> (w5453:T12)
                n2498 = property on="Sampling rate" class="DigNum (strict)"("Visible"=FALSE, "DisabledEnum"=T8."Disabled" ("Disabled")) -> ()  [unwired: 2 in, 2 out]
                n2499 = property on="Pel" class="DigNum (strict)"("Visible"=w5442, "DisabledEnum"=w5443) -> ()  [unwired: 2 in, 2 out]
                n2500 = property on="bin" class="DigNum (strict)"("Visible"=w5442, "DisabledEnum"=w5443) -> ()  [unwired: 2 in, 2 out]
                n2501 = call "2pparameters.vi"("Params in"=w5453, "command"="set") -> ()  [unwired: 1 out]
              }
              frame "Lifetime (point)" {
                w5476 = T8."Enabled" ("Disabled")
                w5475 = TRUE ("Visible")
                n2502 = property on="Pel" class="DigNum (strict)"("Visible"=w5475, "DisabledEnum"=w5476) -> ()  [unwired: 2 in, 2 out]
                n2503 = property on="bin" class="DigNum (strict)"("Visible"=w5475, "DisabledEnum"=w5476) -> ()  [unwired: 2 in, 2 out]
                n2504 = property on="ttt" class="Enum (strict)"("Visible"=FALSE) -> ()  [unwired: 2 in, 2 out]
                n2505 = local write "Zscantab"(enum32{"withzscan", "withoutzscan", "lifetime"}."lifetime" ("Zscantab")) -> ()
                n2506 = local write "graphtab"(T6."Lifetime" ("graphtab")) -> ()
                n2507 = local write "Meastab"(enum32{"X-Y Image", "Linescan", "Timetrace"}."Timetrace" ("Meastab")) -> ()
                n2508 = call "lifetimeparameters.vi"("command"="get") -> ("Params out"=w5483:T21)  [unwired: 1 in]
                n2509 = Unbundle By Name(w5483) -> ("initialized"=w5484:bool)
                n2510 = property on="srateAODOtt" class="DigNum (strict)"("Visible"=TRUE, "DisabledEnum"=T8."Enabled" ("Disabled")) -> ()  [unwired: 2 in, 2 out]
                n2511 = case shown="False" w5484 {
                  frame False {
                    n2512 = property on="Init" class="Bool (strict)"("Visible"=TRUE, "DisabledEnum"=T8."Enabled" ("Disabled")) -> ()  [unwired: 2 in, 2 out]
                    n2513 = property on="Start" class="Bool (strict)"("Visible"=FALSE, "DisabledEnum"=T8."Disabled and Grayed Out" ("Disabled")) -> ()  [unwired: 2 in, 2 out]
                  }
                  frame True {
                  }
                }
                n2514 = property on="Sampling rate" class="DigNum (strict)"("Visible"=FALSE, "DisabledEnum"=T8."Disabled" ("Disabled")) -> ()  [unwired: 2 in, 2 out]
              }
              frame "Lifetime (scan)" {
                w5493 = T8."Disabled" ("Disabled")
                w5492 = FALSE ("Visible")
                n2515 = call "lifetimeparameters.vi"("command"="get") -> ("Params out"=w5505:T21)  [unwired: 1 in]
                n2516 = local write "graphtab"(T6."image" ("graphtab")) -> ()
                n2517 = local write "Save tab"(enum32{"withsave", "withoutsave"}."withsave" ("Save tab")) -> ()
                n2518 = local write "Meastab"(enum32{"X-Y Image", "Linescan", "Timetrace"}."X-Y Image" ("Meastab")) -> ()
                n2519 = local write "Zscantab"(enum32{"withzscan", "withoutzscan", "lifetime"}."lifetime" ("Zscantab")) -> ()
                n2520 = Unbundle By Name(w5505) -> ("initialized"=w5504:bool)
                n2521 = property on="ttt" class="Enum (strict)"("Visible"=FALSE) -> ()  [unwired: 2 in, 2 out]
                n2522 = property on="refreshtime" class="DigNum (strict)"("Visible"=FALSE, "DisabledEnum"=T8."Disabled and Grayed Out" ("Disabled")) -> ()  [unwired: 2 in, 2 out]
                n2523 = property on="Pel" class="DigNum (strict)"("Visible"=w5492, "DisabledEnum"=w5493) -> ()  [unwired: 2 in, 2 out]
                n2524 = property on="bin" class="DigNum (strict)"("Visible"=w5492, "DisabledEnum"=w5493) -> ()  [unwired: 2 in, 2 out]
                n2525 = property on="save data" class="Bool (strict)"("Visible"=TRUE, "DisabledEnum"=T8."Enabled" ("Disabled"), "Value"=TRUE ("Visible")) -> ()  [unwired: 2 in, 2 out]
                n2526 = case shown="False" w5504 {
                  frame False {
                    n2527 = property on="Init" class="Bool (strict)"("Visible"=TRUE, "DisabledEnum"=T8."Enabled" ("Disabled")) -> ()  [unwired: 2 in, 2 out]
                    n2528 = property on="Start" class="Bool (strict)"("Visible"=FALSE, "DisabledEnum"=T8."Disabled and Grayed Out" ("Disabled")) -> ()  [unwired: 2 in, 2 out]
                  }
                  frame True {
                  }
                }
                n2529 = call "2pparameters.vi"("command"="get") -> ("params out"=w5510:T12)  [unwired: 1 in]
                n2530 = property on="continuous" class="Bool (strict)"("Visible"=TRUE, "DisabledEnum"=T8."Disabled and Grayed Out" ("Disabled")) -> ()  [unwired: 2 in, 2 out]
                n2531 = property on="finite samples" class="Bool (strict)"("Visible"=TRUE, "DisabledEnum"=T8."Enabled" ("Disabled")) -> ()  [unwired: 2 in, 2 out]
                n2532 = Bundle By Name(cluster=w5510, "type"="Lifetime (scan)") -> (w5508:T12)
                n2533 = call "2pparameters.vi"("Params in"=w5508, "command"="set") -> ()  [unwired: 1 out]
                n2534 = property on="finite samples" class="Bool (strict)"("Val(Sgnl)"=TRUE ("continuous for display")) -> ()  [unwired: 2 in, 2 out]
                n2535 = property on="continuous" class="Bool (strict)"("Value"=FALSE ("continuous for display")) -> ()  [unwired: 2 in, 2 out]
                n2536 = property on="srateAODOtt" class="DigNum (strict)"("Visible"=FALSE, "DisabledEnum"=T8."Disabled" ("Disabled")) -> ()  [unwired: 2 in, 2 out]
                n2537 = property on="# of frames" class="DigNum (strict)"("DisabledEnum"=T8."Enabled" ("Disabled"), "Caption.Text"="# of frames") -> ()  [unwired: 2 in, 2 out]
                n2538 = property on="img_CH1" class="IntGraph (strict)"("ZScale.Maximum"=12.5 ("Z Scale.Range:Maximum")) -> ()  [unwired: 2 in, 2 out]
                n2539 = property on="Current Average" class="DigNum (strict)"("Visible"=TRUE, "DisabledEnum"=T8."Enabled" ("Disabled")) -> ()  [unwired: 2 in, 2 out]
                n2540 = property on="Sampling rate" class="DigNum (strict)"("Visible"=TRUE, "DisabledEnum"=T8."Enabled" ("Disabled")) -> ()  [unwired: 2 in, 2 out]
                n2541 = property on="avpp" class="DigNum (strict)"("Visible"=TRUE, "DisabledEnum"=T8."Enabled" ("Disabled")) -> ()  [unwired: 2 in, 2 out]
              }
              frame "Lifetime (contour)" {
                w5534 = T8."Enabled" ("Disabled")
                w5533 = TRUE ("Visible")
                n2542 = call "2pparameters.vi"("command"="get") -> ("params out"=w5541:T12)  [unwired: 1 in]
                n2543 = property on="# of frames" class="DigNum (strict)"("DisabledEnum"=T8."Enabled" ("Disabled"), "Caption.Text"="# of samples") -> ()  [unwired: 2 in, 2 out]
                n2544 = property on="refreshtime" class="DigNum (strict)"("Visible"=TRUE, "DisabledEnum"=T8."Enabled" ("Disabled")) -> ()  [unwired: 2 in, 2 out]
                n2545 = Unbundle By Name(w5541) -> ("Angle draw"=w5543:dbl)
                n2546 = property on="avpp" class="DigNum (strict)"("Visible"=FALSE, "DisabledEnum"=T8."Disabled and Grayed Out" ("Disabled")) -> ()  [unwired: 2 in, 2 out]
                n2547 = property on="Current Average" class="DigNum (strict)"("Visible"=FALSE, "DisabledEnum"=T8."Disabled and Grayed Out" ("Disabled")) -> ()  [unwired: 2 in, 2 out]
                n2548 = local write "Angle drawing"(w5543) -> ()
                n2549 = local write "Save tab"(enum32{"withsave", "withoutsave"}."withsave" ("Save tab")) -> ()
                n2550 = local write "Zscantab"(enum32{"withzscan", "withoutzscan", "lifetime"}."lifetime" ("Zscantab")) -> ()
                n2551 = local write "graphtab"(T6."Lifetime" ("graphtab")) -> ()
                n2552 = local write "Meastab"(enum32{"X-Y Image", "Linescan", "Timetrace"}."Timetrace" ("Meastab")) -> ()
                n2553 = property on="ttt" class="Enum (strict)"("Visible"=TRUE) -> ()  [unwired: 2 in, 2 out]
                n2554 = call "lifetimeparameters.vi"("command"="get") -> ("Params out"=w5565:T21)  [unwired: 1 in]
                n2555 = property on="finite samples" class="Bool (strict)"("Val(Sgnl)"=TRUE ("continuous for display")) -> ()  [unwired: 2 in, 2 out]
                n2556 = local write "save\ndata"(TRUE ("save\ndata")) -> ()
                n2557 = Unbundle By Name(w5565) -> ("initialized"=w5566:bool)
                n2558 = property on="continuous" class="Bool (strict)"("Visible"=TRUE, "DisabledEnum"=T8."Enabled" ("Disabled")) -> ()  [unwired: 2 in, 2 out]
                n2559 = property on="finite samples" class="Bool (strict)"("Visible"=TRUE, "DisabledEnum"=T8."Enabled" ("Disabled")) -> ()  [unwired: 2 in, 2 out]
                n2560 = property on="Pel" class="DigNum (strict)"("Visible"=w5533, "DisabledEnum"=w5534) -> ()  [unwired: 2 in, 2 out]
                n2561 = property on="bin" class="DigNum (strict)"("Visible"=w5533, "DisabledEnum"=w5534) -> ()  [unwired: 2 in, 2 out]
                n2562 = property on="continuous" class="Bool (strict)"("Value"=FALSE ("continuous for display")) -> ()  [unwired: 2 in, 2 out]
                n2563 = case shown="False" w5566 {
                  frame False {
                    n2564 = property on="Init" class="Bool (strict)"("Visible"=TRUE, "DisabledEnum"=T8."Enabled" ("Disabled")) -> ()  [unwired: 2 in, 2 out]
                    n2565 = property on="Start" class="Bool (strict)"("Visible"=FALSE, "DisabledEnum"=T8."Disabled and Grayed Out" ("Disabled")) -> ()  [unwired: 2 in, 2 out]
                  }
                  frame True {
                  }
                }
                n2566 = property on="srateAODOtt" class="DigNum (strict)"("Visible"=TRUE, "DisabledEnum"=T8."Enabled" ("Disabled")) -> ()  [unwired: 2 in, 2 out]
                n2567 = call "2pparameters.vi"("command"="get") -> ("params out"=w5545:T12)  [unwired: 1 in]
                n2568 = Bundle By Name(cluster=w5545, "type"="Timetrace") -> (w5539:T12)
                n2569 = call "2pparameters.vi"("Params in"=w5539, "command"="set") -> ()  [unwired: 1 out]
                n2570 = property on="Sampling rate" class="DigNum (strict)"("Visible"=FALSE, "DisabledEnum"=T8."Disabled" ("Disabled")) -> ()  [unwired: 2 in, 2 out]
              }
            }
          }
          event "Laserpower \n(%)": Value Change {
            n2571 = event-data() -> ("OldVal"=w5574:dbl, "NewVal"=w5575:dbl)  [unwired: 1 in, 4 out]
            n2572 = Not Equal?(x=w5574, y=w5575) -> (x != y?=w5576:bool)
            n2573 = case shown="True" w5576 {
              tunnel: w5575 -> [_ w5577]
              frame False {
              }
              frame True {
                n2574 = local read "wavelength(nm)"() -> (w5579:dbl)
                n2575 = call "configuration.vi"("command"="get") -> ("config out"=w5583:T13)  [unwired: 2 in, 1 out]
                n2576 = call "pockelscellcalibration.vi"("l"=w5579, "T"=w5577) -> ("Vout"=w5578:dbl)
                n2577 = Unbundle By Name(w5583) -> ("Vto2P"=w5582:i32, "AOlines"=w5581:tag[])
                n2578 = property on="lpow" class="DigNum (strict)"("Value"=w5577) -> ()  [unwired: 2 in, 2 out]
                n2579 = Index Array(array=w5581, index=w5582) -> (element=w5580:tag)
                n2580 = call-poly <vilib>:"DAQmx Create Virtual Channel.vi"("physical channels"=w5580) -> ("task out"=w5586:refnum<k21>, "error out"=w5585:errorcluster)  [unwired: 13 in]
                n2581 = call-poly <vilib>:"DAQmx Write.vi"("task/channels in"=w5586, "data"=w5578, "error in"=w5585) -> ("task out"=w5587:refnum<k21>, "error out"=w5588:errorcluster)  [unwired: 10 in, 1 out]
                n2582 = call <vilib>:"DAQmx Start Task.vi"("task/channels in"=w5587, "error in"=w5588) -> ("task out"=w5589:refnum<k21>, "error out"=w5590:errorcluster)  [unwired: 12 in]
                n2583 = call <vilib>:"DAQmx Stop Task.vi"("task/channels in"=w5589, "error in"=w5590) -> ("task out"=w5591:refnum<k21>, "error out"=w5592:errorcluster)  [unwired: 12 in]
                n2584 = call <vilib>:"DAQmx Clear Task.vi"("task in"=w5591, "error in"=w5592) -> ()  [unwired: 13 in, 1 out]
              }
            }
          }
          event "lpow": Value Change {
            n2585 = event-data() -> ("OldVal"=w5593:dbl, "NewVal"=w5594:dbl)  [unwired: 1 in, 4 out]
            n2586 = Not Equal?(x=w5593, y=w5594) -> (x != y?=w5595:bool)
            n2587 = case shown="True" w5595 {
              tunnel: w5594 -> [_ w5598]
              frame False {
              }
              frame True {
                n2588 = local read "wavelength(nm)"() -> (w5597:dbl)
                n2589 = call "pockelscellcalibration.vi"("l"=w5597, "T"=w5598) -> ("Vout"=w5596:dbl)
                n2590 = call "configuration.vi"("command"="get") -> ("config out"=w5602:T13)  [unwired: 2 in, 1 out]
                n2591 = Unbundle By Name(w5602) -> ("Vto2P"=w5601:i32, "AOlines"=w5600:tag[])
                n2592 = property on="Laserpower \n(%)" class="Slide (strict)"("Value"=w5598) -> ()  [unwired: 2 in, 2 out]
                n2593 = Index Array(array=w5600, index=w5601) -> (element=w5599:tag)
                n2594 = call-poly <vilib>:"DAQmx Create Virtual Channel.vi"("physical channels"=w5599) -> ("task out"=w5605:refnum<k21>, "error out"=w5604:errorcluster)  [unwired: 13 in]
